vi "Write Choice.vi"(8 "error in (no error)":errorcluster, 10 "Choice":bool, 11 "_Popup in":refnum<class "Popup.lvclass">) -> (0 "error out":errorcluster, 3 "_Popup out":refnum<class "Popup.lvclass">)   [LabVIEW 2021, in "Pop-Up.lvlib" / "Popup.lvclass"]
doc: "This Data Member Access VI will write the Choice Boolean to the object.\n\nInputs: +\n-Choice [Boolean] - the value to write to the object\n\n<b>Code Developed By:</b> +\nDaniel Coons +\nhttps://github.com/danielcoons/tsc-pop-up"
uses:
  Popup.lvclass
  Popup.lvclass/Popup.ctl
panel:
  # "This VI puts the choice value (boolean) into the Popup Object"
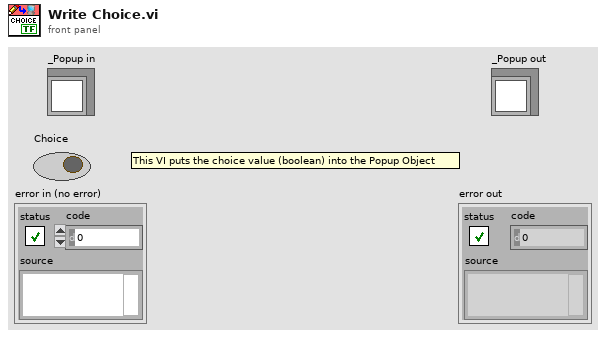
[diagram p1: front panel]
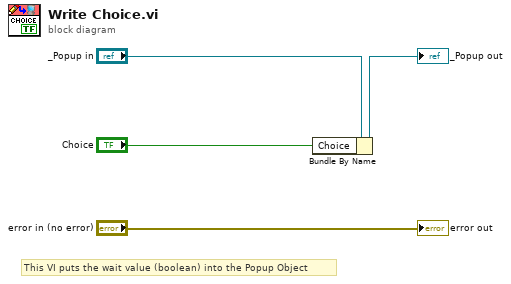
[diagram p0: block diagram]
diagram:
  # "This VI puts the wait value (boolean) into the Popup Object"
  n1 = Bundle By Name(cluster="_Popup in", "Choice"="Choice") -> (→"_Popup out":refnum<class "Popup.lvclass">)
  "error out" <- "error in (no error)"
